vi "Configure Trigger Holdoff.vi"(7 "Enable Trigger Holdoff (F: Disable)":bool, 8 "error in (no error)":errorcluster, 10 "Trigger Holdoff Time (0.1 s)":dbl=0.1, 11 "VISA resource name":refnum<visa-resource-name>) -> (0 "error out":errorcluster, 3 "VISA resource name out":refnum<visa-resource-name>)   [LabVIEW 2014, in "Agilent MXA Series.lvlib"]
doc: "Configures Trigger Holdoff characteristics."
uses:
  Agilent MXA Series.lvlib
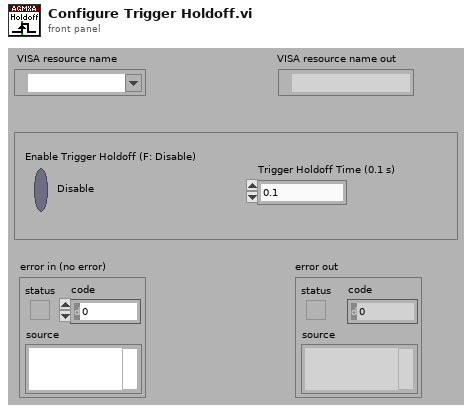
[diagram p1: front panel]
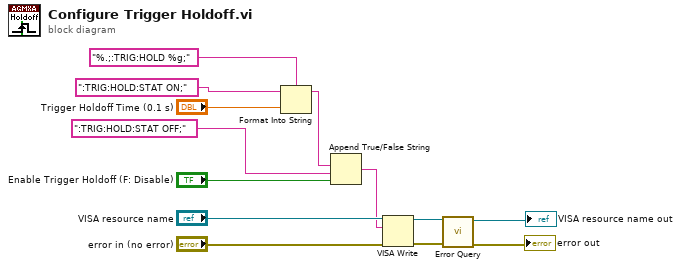
[diagram p0: block diagram]
diagram:
  n1 = Format Into String(format string="%.;:TRIG:HOLD %g;", initial string=":TRIG:HOLD:STAT ON;", "Trigger Holdoff Time (0.1 s)") -> (resulting string=w3:string)  [unwired: 1 in, 1 out]
  n2 = Append True/False String(1:"Enable Trigger Holdoff (F: Disable)", 2:":TRIG:HOLD:STAT OFF;" ("false string"), 3:w3) -> (0:w2:string)  [unwired: 1 in]
  n3 = VISA Write(VISA resource name="VISA resource name", write buffer=w2, error in (no error)="error in (no error)") -> (VISA resource name out=w7:refnum<visa-resource-name>, error out=w6:errorcluster)  [unwired: 1 out]
  n4 = call "Error Query.vi"("error in (no error)"=w6, "VISA resource name"=w7) -> ("error out"=→"error out":errorcluster, "VISA resource name out"=→"VISA resource name out":refnum<visa-resource-name>)  [unwired: 6 in, 2 out]
